vi "diskdriveinfo.vi"(0 "Drive Letter":string, 11 "error in (no error)":errorcluster) -> (1 "Windows error":i32, 2 "root path name":string, 3 "drive name":string, 4 "flags":i32, 6 "file system name":string, 8 "file system name size":i32, 12 "drive name size":i16, 13 "serial number":i32, 14 "max path item length":i32, 15 "error out":errorcluster)   [LabVIEW 2014]
doc: "Windows) Use this VI to retrieve descriptive information, including the serial number, file system, and volume name, for hard drives or disk drives. This VI uses the Call Library Function Node to call the GetVolumeInformation function. Refer to the Microsoft Developer Network Web site at www.msdn.microsoft.com for more information about the GetVolumeInformation function.\n\nNote: LabVIEW might prompt you to open the kernel32 DLL when you open this VI. You can find the kernel32 DLL in the WINDOWS\\SYSTEM32 directory. On the block diagram, double-click the Call Library Function Node and click the Browse button to navigate to the correct DLL."
uses:
  C:/Windows/System32/kernel32.dll
panel:
  in  "lpFilesystemNameBuffer":string="0000000000000                   0000000000000000000000000000000000000000000000000000000000000000000000000000000000000000000000000000000000000000000000000000000000000000000000000000000000000000000000000000000000000000000000000000000000000000000000000000000"
  in  "lpVolumeNameBuffer_input":string="0000000000000                   0000000000000000000000000000000000000000000000000000000000000000000000000000000000000000000000000000000000000000000000000000000000000000000000000000000000000000000000000000000000000000000000000000000000000000000000000000000"
  # "Select Help»Show Context Help and move the cursor over the VI icon to display help for this VI."
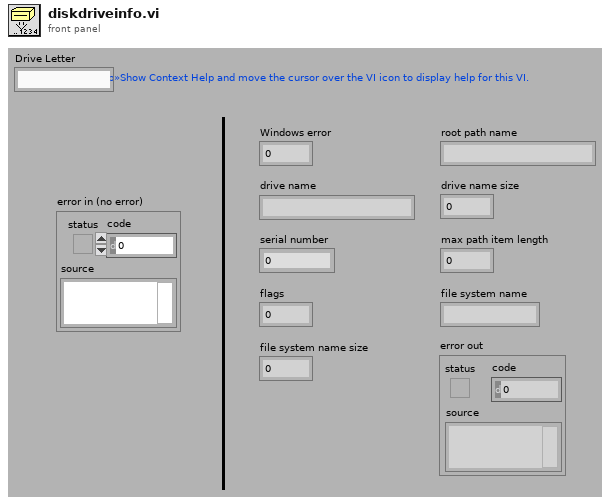
[diagram p1: front panel]
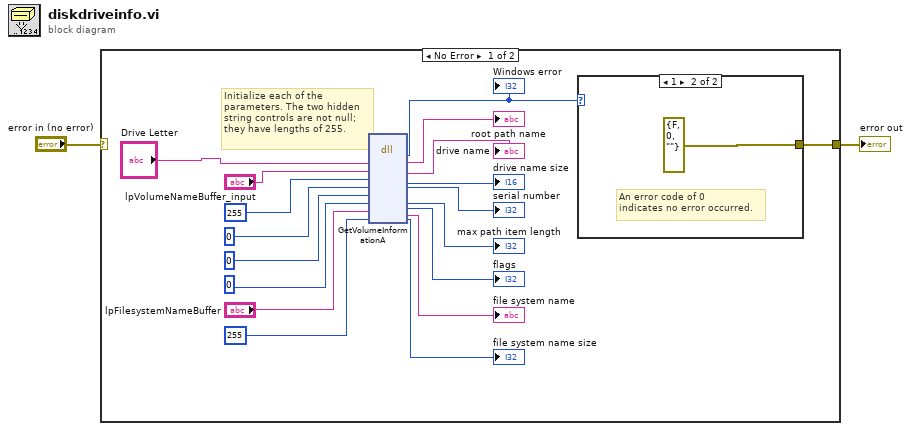
[diagram p0: block diagram]
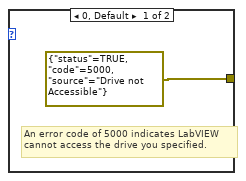
[diagram p2: hidden frame]
diagram:
  n1 = case shown="No Error" "error in (no error)" {
    selector: "error in (no error)" -> [_ w23]
    tunnel: [w5 w23] -> w1
    frame No Error {
      # "Initialize each of the\nparameters. The two hidden\nstring controls are not null;\nthey have lengths of 255."
      n2 = dll-call lib="C:/Windows/System32/kernel32.dll" fn="GetVolumeInformationA"("lpRootPathName"="Drive Letter", "lpVolumeNameBuffer"="lpVolumeNameBuffer_input", "nVolumeNameSize"=i16 255, "lpVolumeSerialNumber"=0, "lpMaximumComponentLength"=0, "lpFileSystemFlags"=0, "lpFileSystemNameBuffer"="lpFilesystemNameBuffer", "nFileSystemNameSize"=255) -> ("return type"=w20:i32, "lpRootPathName"=→"root path name":string, "lpVolumeNameBuffer"=→"drive name":string, "nVolumeNameSize"=→"drive name size":i16, "lpVolumeSerialNumber"=→"serial number":i32, "lpMaximumComponentLength"=→"max path item length":i32, "lpFileSystemFlags"=→"flags":i32, "lpFileSystemNameBuffer"=→"file system name":string, "nFileSystemNameSize"=→"file system name size":i32)  [unwired: 3 in, 2 out]
      "Windows error" <- w20
      n3 = case shown="1" w20 {
        tunnel: [errorcluster {"status"=TRUE, "code"=5000, "source"="Drive not Accessible"} ("error out") errorcluster {"status"=FALSE, "code"=0, "source"=""} ("error out")] -> w5
        frame 0, Default {
          # "An error code of 5000 indicates LabVIEW\ncannot access the drive you specified."
        }
        frame 1 {
          # "An error code of 0\nindicates no error occurred."
        }
      }
    }
    frame Error {
    }
  }
  "error out" <- w1
